vi "Caps_pressure_discharge.vi"() -> ()   [LabVIEW 2011]
panel:
  out "timing (ns) 2":dbl
  in  "timing (ns)":dbl
  out "x 4":dbl
  out "x 3":dbl
  in  "x 2":dbl
  in  "x":dbl
  in  "discharge2::4":bool caption="CAP2"
  in  "discharge1::4":bool caption="CAP1"
  out "discharge 4":dbl
  in  "discharge 3":dbl
  out "discharge 2":dbl
  in  "discharge":dbl
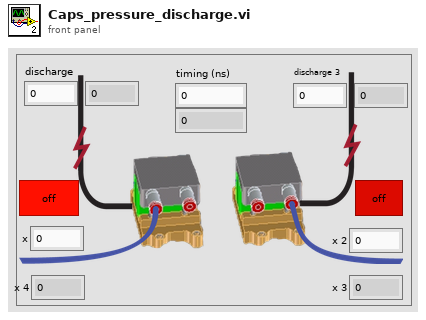
[diagram p1: front panel]
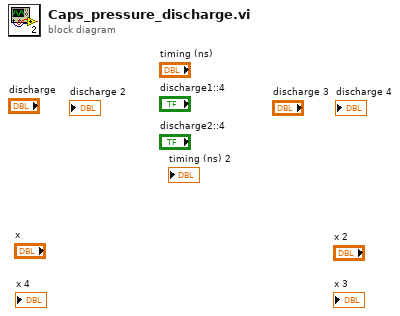
[diagram p0: block diagram]
diagram:
